vi "Trigger Detector (Waveform).vi"(0 "waveforms":waveform(dbl)[](array[waveform]), 1 "reset? (F)":bool, 5 "triggers definition":T3(array[cluster]), 11 "error in (no error)":errorcluster) -> (4 "triggers":T2(array[cluster]), 6 "actual trigger state":T1[](array[typedef]), 15 "error out":errorcluster)   [LabVIEW 2014, in "NI_EP_Power Quality.lvlib"]
doc: "Detects crossing of limits for the measurement that you specify and returns triggers if occur.\n\nThis VI supports measuring single-line and multiple-line systems except the DBL instance. Use the DBL instance to measure one channel on one line at one time."
uses:
  <vilib>/addons/Electrical Power/PQ/NI_EP_Power Quality.lvlib
  <vilib>/addons/Electrical Power/PQ/Common/Controls/ep_Trigger State.ctl
  <vilib>/addons/Electrical Power/PQ/Triggers/subVIs/ep_Trigger Definition.ctl
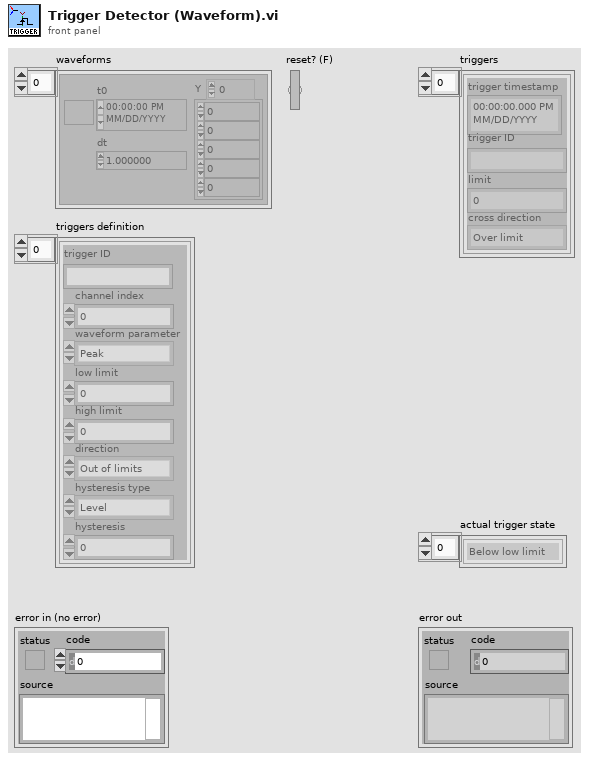
[diagram p1: front panel]
types:
  T1 = typedef "NI_EP_Power Quality.lvlib/ep_Trigger State.ctl" = enum16{"Below low limit", "In the limits", "Over high limit"}
  T2 = cluster{"trigger timestamp":timestamp, "trigger ID":string, "limit":dbl, "cross direction":enum16{"Over limit", "Below limit"}}[]
  T3 = cluster{"trigger ID":string, "channel index":u32, "waveform parameter":enum16{"Peak", "Rate of rise (d/dt)"}, "low limit":dbl, "high limit":dbl, "direction":enum16{"Out of limits", "Back to limits", "Both"}, "hysteresis type":enum16{"Level", "Time"}, "hysteresis":dbl}[]
  T4 = cluster{"trigger time":timestamp, "trigger unique id":string, "limit":dbl, "cross direction":enum16{"Over limit", "Below limit"}}[]
  T5 = typedef "NI_EP_Power Quality.lvlib/ep_Trigger Definition.ctl" = cluster{"trigger ID":string, "low limit":dbl, "high limit":dbl, "direction":enum16{"Out of limits", "Back to limits", "Both"}, "hysteresis type":enum16{"Level", "Time"}, "hysteresis":dbl}
  T6 = cluster{"Lo in progr.":bool, "Lo in progr.":bool, "t0":timestamp, "t0":timestamp}[]
  T7 = enum16{"Out of limits", "Back to limits", "Both"}
  T8 = cluster{"Lo in progr.":bool, "Lo in progr.":bool, "t0":timestamp, "t0":timestamp}
  T9 = cluster{"Lo in progr.":bool, "Hi in progr.":bool, "Lo trig. time":timestamp, "Hi trig. time":timestamp}
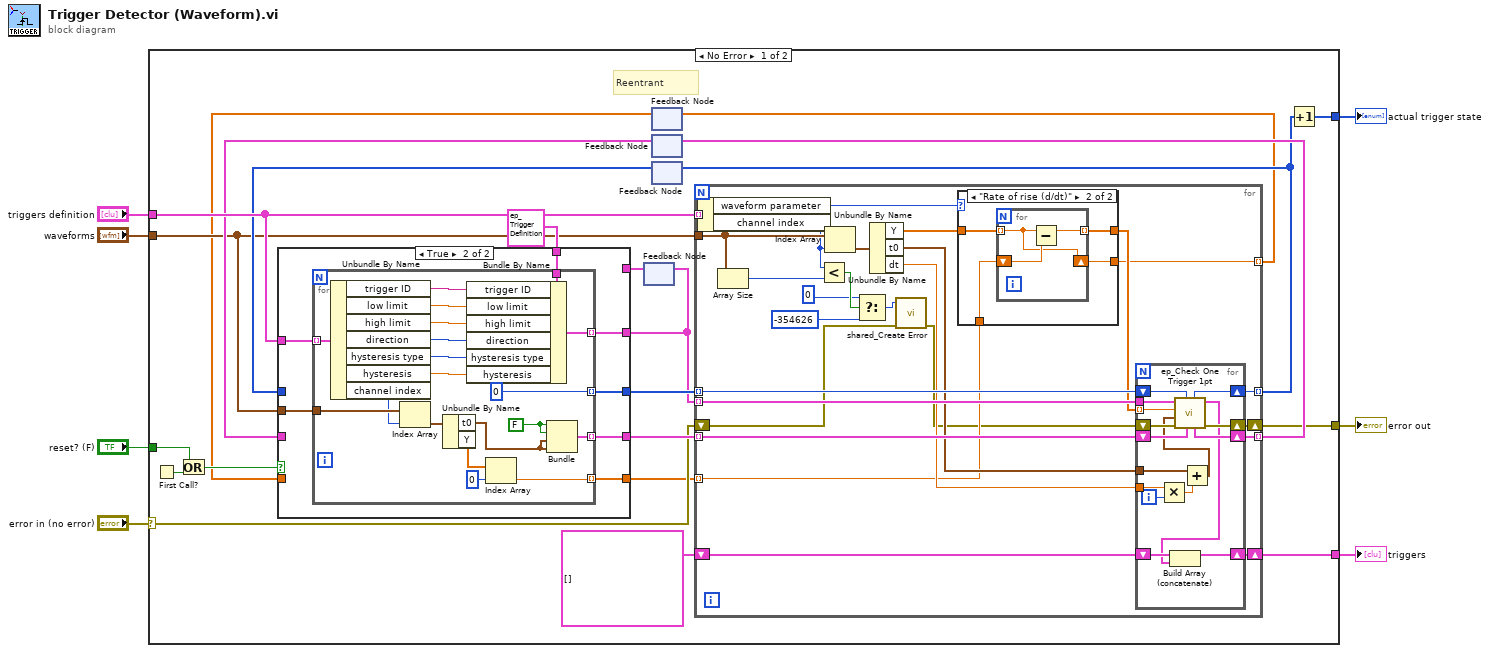
[diagram p0: block diagram]
diagram:
  n1 = case shown="No Error" "error in (no error)" {
    selector: "error in (no error)" -> [w13 w111]
    tunnel: "waveforms" -> [w14 _]
    tunnel: "reset? (F)" -> [w28 _]
    tunnel: "triggers definition" -> [w26 _]
    tunnel: [w16 _] -> w6
    tunnel: [w15 w111] -> w7
    tunnel: [w11 _] -> w1
    frame No Error {
      # "Reentrant"
      n2 = First Call?() -> (First Call?: T/F=w29:bool)
      n3 = Or(x=w28, y=w29) -> (x .or. y?=w27:bool)
      n4 = feedback #1() -> (w19:T5[])  [unwired: 1 in]
      n5 = feedback #2() -> (w8:dbl[])  [unwired: 1 in]
      n6 = feedback #3() -> (w20:T6)  [unwired: 1 in]
      n7 = feedback #4() -> (w22:i8[])  [unwired: 1 in]
      n8 = case shown="True" w27 {
        tunnel: w26 -> [_ w40]
        tunnel: [w31 w39] -> w18
        tunnel: T5 {"trigger ID"="", "low limit"=0.0, "high limit"=0.0, "direction"=enum."Out of limits", "hysteresis type"=enum."Level", "hysteresis"=0.0} ("trigger definition") -> [_ w38]
        tunnel: [w33 w37] -> w24
        tunnel: [w32 w36] -> w23
        tunnel: w22 -> [w32 _]
        tunnel: w20 -> [w33 _]
        tunnel: w19 -> [w31 _]
        tunnel: w14 -> [_ w35]
        tunnel: [w30 w34] -> w10
        tunnel: w8 -> [w30 _]
        frame False {
        }
        frame True {
          n9 = for {
            tunnel: w40 -> [w55] mode=indexing
            tunnel: [w54] -> w39 mode=indexing
            tunnel: w38 -> [w53]
            tunnel: [w50] -> w37 mode=indexing
            tunnel: [i8 0] -> w36 mode=indexing
            tunnel: w35 -> [w47]
            tunnel: [w41] -> w34 mode=indexing
            w51 = FALSE ("Lo in progr.")
            n10 = Unbundle By Name(w55) -> ("trigger ID"=w58:string, "low limit"=w49:dbl, "high limit"=w48:dbl, "direction"=w57:T7, "hysteresis type"=w56:enum16{"Level", "Time"}, "hysteresis"=w59:dbl, "channel index"=w46:u32)
            n11 = Index Array(array=w47, index=w46) -> (element=w45:waveform(dbl))
            n12 = Unbundle By Name(w45) -> ("t0"=w44:timestamp, "Y"=w43:dbl[])
            n13 = Bundle By Name(cluster=w53, "trigger ID"=w58, "low limit"=w49, "high limit"=w48, "direction"=w57, "hysteresis type"=w56, "hysteresis"=w59) -> (w54:T5)
            n14 = Index Array(array=w43, index=0) -> (element=w41:dbl)
            n15 = Bundle("Lo in progr."=w51, "Lo in progr."=w51, "t0"=w44, "t0"=w44) -> (w50:T8)  [unwired: 1 in]
          }
        }
      }
      n16 = feedback-in #1(w18) -> ()
      n17 = for {
        tunnel: w26 -> [w81] mode=indexing
        tunnel: w14 -> [w78]
        tunnel: w24 -> [w80] mode=indexing
        tunnel: w23 -> [w84] mode=indexing
        tunnel: [w83] -> w12 mode=indexing
        tunnel: [w82] -> w21 mode=indexing
        tunnel: w18 -> [w85] mode=indexing
        shift-right: [w73] -> w16
        shift-left: T4 [] -> [w74]
        shift-right: [w79] -> w15
        shift-left: w13 -> [w61]
        tunnel: w10 -> [w66] mode=indexing
        tunnel: [w65] -> w9 mode=indexing
        n18 = Unbundle By Name(w81) -> ("waveform parameter"=w69:enum16{"Peak", "Rate of rise (d/dt)"}, "channel index"=w77:u32)
        n19 = Array Size(array=w78) -> (size(s)=w76:i32)
        n20 = Less?(x=w77, y=w76) -> (x < y?=w75:bool)
        n21 = Index Array(array=w78, index=w77) -> (element=w72:waveform(dbl))
        n22 = Select(t=0 ("error code (0)"), s=w75, f=-354626 ("error code (0)")) -> (s? t:f=w62:i32)
        n23 = Unbundle By Name(w72) -> ("Y"=w68:dbl[], "t0"=w71:timestamp, "dt"=w70:dbl)
        n24 = call <vilib>:"shared_Create Error.vi"("error in (no error)"=w61, "error code (0)"=w62) -> ("error out"=w60:errorcluster)  [unwired: 9 in]
        n25 = case shown="\"Rate of rise (d/dt)\"" w69 {
          tunnel: w68 -> [w87 w91]
          tunnel: [w87 w90] -> w67
          tunnel: w66 -> [w86 w89]
          tunnel: [w86 w88] -> w65
          frame "Peak", Default {
          }
          frame "Rate of rise (d/dt)" {
            n26 = for {
              tunnel: w91 -> [w92] mode=indexing
              shift-right: [w92] -> w88
              shift-left: w89 -> [w94]
              tunnel: [w93] -> w90 mode=indexing
              n27 = Subtract(x=w92, y=w94) -> (x-y=w93:dbl)
            }
          }
        }
        n28 = for {
          tunnel: w85 -> [w110]
          shift-right: [w108] -> w83
          shift-left: w84 -> [w109]
          shift-right: [w105] -> w79
          shift-left: w60 -> [w104]
          shift-right: [w107] -> w82
          shift-left: w80 -> [w106]
          shift-right: [w101] -> w73
          shift-left: w74 -> [w103]
          tunnel: w67 -> [w100] mode=indexing
          tunnel: w71 -> [w97]
          tunnel: w70 -> [w98]
          i -> [w99]
          n29 = Multiply(x=w98, y=w99) -> (x*y=w96:dbl)
          n30 = Add(x=w97, y=w96) -> (x+y=w95:timestamp)
          n31 = call <vilib>:"ep_Check One Trigger 1pt.vi"("trig. local in"=w106, "prev. state in"=w109, "error in (no error)"=w104, "data time stamp"=w95, "value in"=w100, "trigger definition"=w110) -> ("error out"=w105:errorcluster, "triggers list"=w102:T4, "trig. local out"=w107:T9, "state out"=w108:i8)  [unwired: 2 in]
          n32 = Build Array (concatenate)(w103, w102) -> (w101:T4)
        }
      }
      n33 = feedback-in #2(w9) -> ()
      n34 = feedback-in #3(w21) -> ()
      n35 = feedback-in #4(w12) -> ()
      n36 = Increment(x=w12) -> (x+1=w11:i8[])
    }
    frame Error {
    }
  }
  "error out" <- w7
  "triggers" <- w6
  "actual trigger state" <- w1
